vi "GetTestMap.vi"(8 "error in (no error)":errorcluster, 11 "ResultTreeListener in":refnum<class "ResultTreeListener.lvclass">) -> (0 "error out":errorcluster, 2 "Test Map":T1(array[cluster]), 3 "ResultTreeListener out":refnum<class "ResultTreeListener.lvclass">)   [LabVIEW 2017, in "ResultTreeListener.lvclass"]
doc: "Returns a map of tags and tests."
uses:
  ResultTreeListener.lvclass
  Test/Test.lvclass
  ResultTreeListener.lvclass/ResultTreeListener.ctl
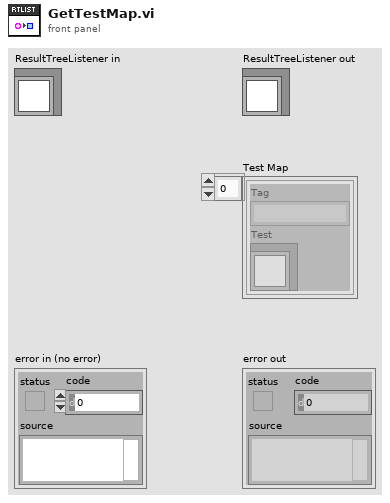
[diagram p1: front panel]
types:
  T1 = cluster{"Tag":string, "Test":refnum<class "Test.lvclass">}[]
  T2 = cluster{"Tag":string, "Test":refnum<class "Test.lvclass">}
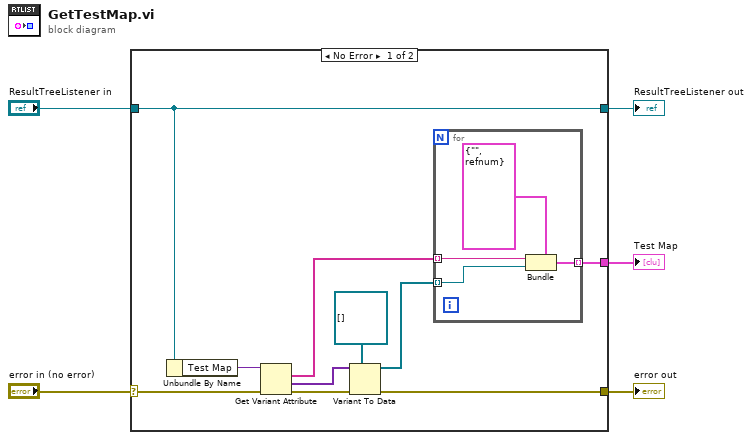
[diagram p0: block diagram]
diagram:
  n1 = case shown="No Error" "error in (no error)" {
    selector: "error in (no error)" -> [w13 w21]
    tunnel: [w11 w21] -> w4
    tunnel: [w15 w20] -> w2
    tunnel: "ResultTreeListener in" -> [w15 w20]
    tunnel: [w6 _] -> w1
    frame No Error {
      n2 = Unbundle By Name(w15) -> ("Test Map"=w14:variant)
      n3 = Get Variant Attribute(Variant=w14, error in=w13) -> (names=w8:string[], values=w10:variant[], error out=w12:errorcluster)  [unwired: 2 in, 1 out]
      n4 = Variant To Data(error in=w12, type=refnum<class "Test.lvclass">[] [] ("Array"), Variant=w10) -> (data=w7:refnum<class "Test.lvclass">[], error out=w11:errorcluster)
      n5 = for {
        tunnel: w8 -> [w19] mode=indexing
        tunnel: w7 -> [w18] mode=indexing
        tunnel: [w16] -> w6 mode=indexing
        n6 = Bundle(cluster=T2 {"Tag"="", "Test"=refnum}, "Tag"=w19, "Test"=w18) -> (w16:T2)
      }
    }
    frame Error {
    }
  }
  "error out" <- w4
  "ResultTreeListener out" <- w2
  "Test Map" <- w1
